vi "LH_InsertAheadIndex.vi"(1 "Index":i32, 2 "InsertContent":i32, 3 "InputList":refnum<class "ListHead.lvclass">) -> (0 "OutputList":refnum<class "ListHead.lvclass">)   [LabVIEW 2014, in "ListHead.lvclass"]
uses:
  ListHead.lvclass
  ListHead.lvclass/ListHead.ctl
  ListNode.lvclass
  ListNodeVirtual.lvclass
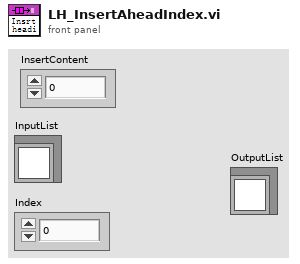
[diagram p1: front panel]
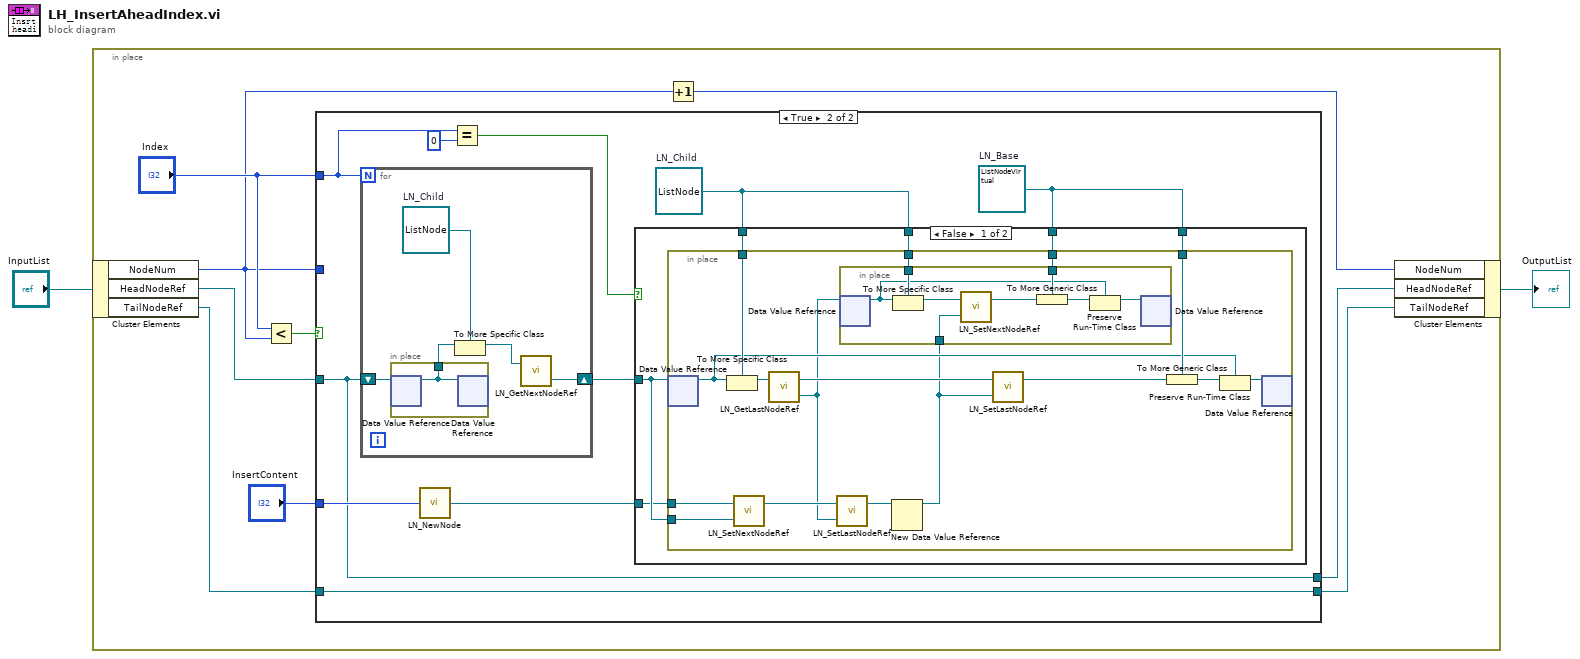
[diagram p0: block diagram]
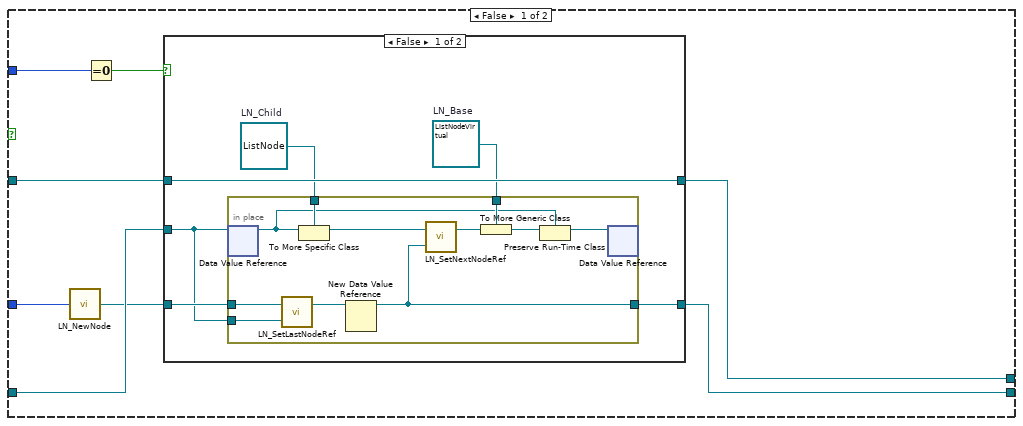
[diagram p2: hidden frame]
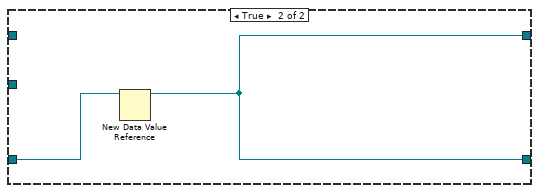
[diagram p3: hidden frame]
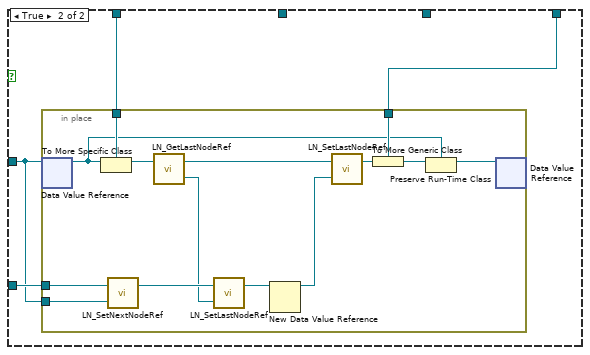
[diagram p4: hidden frame]
diagram:
  n1 = in-place {
    n2 = in-place-cluster #1("InputList") -> ("NodeNum"=w3:u32, "HeadNodeRef"=w9:refnum<data-value>, "TailNodeRef"=w8:refnum<data-value>)
    n3 = Less?(x="Index", y=w3) -> (x < y?=w10:bool)
    n4 = case shown="True" w10 {
      tunnel: w9 -> [w17 w45]
      tunnel: "Index" -> [_ w43]
      tunnel: "InsertContent" -> [w15 w48]
      tunnel: w8 -> [w16 w44]
      tunnel: [w13 w45] -> w5
      tunnel: [w12 w44] -> w4
      tunnel: w3 -> [w19 _]
      frame False {
        n5 = call "LN_NewNode.vi"("InputContent"=w15) -> ("OutputListNode"=w14:refnum<class "ListNode.lvclass">)
        n6 = Equal To 0?(x=w19) -> (x = 0?=w18:bool)
        n7 = case shown="False" w18 {
          tunnel: w14 -> [w23 w38]
          tunnel: w17 -> [w25 _]
          tunnel: w16 -> [w22 _]
          tunnel: [w20 w37] -> w12
          tunnel: [w25 w37] -> w13
          frame False {
            w21 = refnum<class "ListNodeVirtual.lvclass"> refnum  # LN_Base
            w24 = refnum<class "ListNode.lvclass"> refnum  # LN_Child
            n8 = in-place {
              in-place-border: [w27] -> w20
              in-place-border: w24 -> [w36]
              in-place-border: w23 -> [w31]
              in-place-border: w22 -> [w30]
              in-place-border: w21 -> [w35]
              n9 = in-place-dvr #2(w22) -> (w33:refnum<class "ListNodeVirtual.lvclass">)  [unwired: 1 out]
              n10 = call "LN_SetLastNodeRef.vi"("InputLastNodeRef"=w30, "InputListNode"=w31) -> ("OutputListNode"=w29:refnum<class "ListNode.lvclass">)  [unwired: 1 in]
              n11 = To More Specific Class(target class=w36, reference=w33) -> (specific class reference=w28:refnum<class "ListNode.lvclass">)  [unwired: 1 in, 1 out]
              n12 = New Data Value Reference(data value=w29) -> (data value reference=w27:refnum<data-value>)  [unwired: 1 in, 1 out]
              n13 = call "LN_SetNextNodeRef.vi"("InputNextNodeRef"=w27, "InputListNode"=w28) -> ("OutputListNode"=w26:refnum<class "ListNode.lvclass">)  [unwired: 1 in]
              n14 = To More Generic Class(target class=w35, reference=w26) -> (generic class reference=w34:refnum<class "ListNodeVirtual.lvclass">)
              n15 = Preserve Run-Time Class(object in=w34, 2:w33) -> (object out=w32:refnum<class "ListNodeVirtual.lvclass">)  [unwired: 1 in, 1 out]
              n16 = in-place-dvr #2(w32) -> ()  [unwired: 2 out]
            }
          }
          frame True {
            n17 = New Data Value Reference(data value=w38) -> (data value reference=w37:refnum<data-value>)  [unwired: 1 in, 1 out]
          }
        }
      }
      frame True {
        w39 = refnum<class "ListNodeVirtual.lvclass"> refnum  # LN_Base
        w40 = refnum<class "ListNode.lvclass"> refnum  # LN_Child
        n18 = for {
          N: w43 -> [_]
          shift-right: [w97] -> w46
          shift-left: w45 -> [w101]
          w100 = refnum<class "ListNode.lvclass"> refnum  # LN_Child
          n19 = in-place {
            in-place-border: [w102] -> w99
            n20 = in-place-dvr #3(w101) -> (w102:refnum<class "ListNodeVirtual.lvclass">)  [unwired: 1 out]
            n21 = in-place-dvr #3(w102) -> ()  [unwired: 2 out]
          }
          n22 = To More Specific Class(target class=w100, reference=w99) -> (specific class reference=w98:refnum<class "ListNode.lvclass">)  [unwired: 1 in, 1 out]
          n23 = call "LN_GetNextNodeRef.vi"("InputListNode"=w98) -> ("OutputNextNodeRef"=w97:refnum<data-value>)  [unwired: 1 in, 1 out]
        }
        n24 = call "LN_NewNode.vi"("InputContent"=w48) -> ("OutputListNode"=w47:refnum<class "ListNode.lvclass">)
        n25 = Equal?(x=w43, y=0) -> (x = y?=w41:bool)
        n26 = case shown="False" w41 {
          tunnel: w40 -> [w52 w82]
          tunnel: w47 -> [w53 w81]
          tunnel: w46 -> [w54 w80]
          tunnel: w39 -> [w51 w79]
          tunnel: w40 -> [w50 _]
          tunnel: w39 -> [w49 _]
          frame False {
            n27 = in-place {
              in-place-border: w52 -> [w70]
              in-place-border: w53 -> [w62]
              in-place-border: w54 -> [w61]
              in-place-border: w51 -> [w69]
              in-place-border: w50 -> [w57]
              in-place-border: w49 -> [w55]
              n28 = in-place-dvr #4(w54) -> (w67:refnum<class "ListNodeVirtual.lvclass">)  [unwired: 1 out]
              n29 = To More Specific Class(target class=w70, reference=w67) -> (specific class reference=w65:refnum<class "ListNode.lvclass">)  [unwired: 1 in, 1 out]
              n30 = call "LN_SetNextNodeRef.vi"("InputNextNodeRef"=w61, "InputListNode"=w62) -> ("OutputListNode"=w60:refnum<class "ListNode.lvclass">)  [unwired: 1 in]
              n31 = call "LN_GetLastNodeRef.vi"("InputListNode"=w65) -> ("OutputLastNodeRef"=w58:refnum<data-value>, "OutputListNode"=w64:refnum<class "ListNode.lvclass">)  [unwired: 1 in]
              n32 = call "LN_SetLastNodeRef.vi"("InputLastNodeRef"=w58, "InputListNode"=w60) -> ("OutputListNode"=w59:refnum<class "ListNode.lvclass">)  [unwired: 1 in]
              n33 = New Data Value Reference(data value=w59) -> (data value reference=w56:refnum<data-value>)  [unwired: 1 in, 1 out]
              n34 = in-place {
                in-place-border: w57 -> [w77]
                in-place-border: w56 -> [w76]
                in-place-border: w55 -> [w74]
                n35 = in-place-dvr #5(w58) -> (w72:refnum<class "ListNodeVirtual.lvclass">)  [unwired: 1 out]
                n36 = To More Specific Class(target class=w77, reference=w72) -> (specific class reference=w78:refnum<class "ListNode.lvclass">)  [unwired: 1 in, 1 out]
                n37 = call "LN_SetNextNodeRef.vi"("InputNextNodeRef"=w76, "InputListNode"=w78) -> ("OutputListNode"=w75:refnum<class "ListNode.lvclass">)  [unwired: 1 in]
                n38 = To More Generic Class(target class=w74, reference=w75) -> (generic class reference=w73:refnum<class "ListNodeVirtual.lvclass">)
                n39 = Preserve Run-Time Class(object in=w73, 2:w72) -> (object out=w71:refnum<class "ListNodeVirtual.lvclass">)  [unwired: 1 in, 1 out]
                n40 = in-place-dvr #5(w71) -> ()  [unwired: 2 out]
              }
              n41 = call "LN_SetLastNodeRef.vi"("InputLastNodeRef"=w56, "InputListNode"=w64) -> ("OutputListNode"=w63:refnum<class "ListNode.lvclass">)  [unwired: 1 in]
              n42 = To More Generic Class(target class=w69, reference=w63) -> (generic class reference=w68:refnum<class "ListNodeVirtual.lvclass">)
              n43 = Preserve Run-Time Class(object in=w68, 2:w67) -> (object out=w66:refnum<class "ListNodeVirtual.lvclass">)  [unwired: 1 in, 1 out]
              n44 = in-place-dvr #4(w66) -> ()  [unwired: 2 out]
            }
          }
          frame True {
            n45 = in-place {
              in-place-border: w82 -> [w96]
              in-place-border: w81 -> [w87]
              in-place-border: w80 -> [w86]
              in-place-border: w79 -> [w95]
              n46 = in-place-dvr #6(w80) -> (w93:refnum<class "ListNodeVirtual.lvclass">)  [unwired: 1 out]
              n47 = To More Specific Class(target class=w96, reference=w93) -> (specific class reference=w91:refnum<class "ListNode.lvclass">)  [unwired: 1 in, 1 out]
              n48 = call "LN_SetNextNodeRef.vi"("InputNextNodeRef"=w86, "InputListNode"=w87) -> ("OutputListNode"=w85:refnum<class "ListNode.lvclass">)  [unwired: 1 in]
              n49 = call "LN_GetLastNodeRef.vi"("InputListNode"=w91) -> ("OutputLastNodeRef"=w84:refnum<data-value>, "OutputListNode"=w90:refnum<class "ListNode.lvclass">)  [unwired: 1 in]
              n50 = call "LN_SetLastNodeRef.vi"("InputLastNodeRef"=w84, "InputListNode"=w85) -> ("OutputListNode"=w83:refnum<class "ListNode.lvclass">)  [unwired: 1 in]
              n51 = New Data Value Reference(data value=w83) -> (data value reference=w88:refnum<data-value>)  [unwired: 1 in, 1 out]
              n52 = call "LN_SetLastNodeRef.vi"("InputLastNodeRef"=w88, "InputListNode"=w90) -> ("OutputListNode"=w89:refnum<class "ListNode.lvclass">)  [unwired: 1 in]
              n53 = To More Generic Class(target class=w95, reference=w89) -> (generic class reference=w94:refnum<class "ListNodeVirtual.lvclass">)
              n54 = Preserve Run-Time Class(object in=w94, 2:w93) -> (object out=w92:refnum<class "ListNodeVirtual.lvclass">)  [unwired: 1 in, 1 out]
              n55 = in-place-dvr #6(w92) -> ()  [unwired: 2 out]
            }
          }
        }
      }
    }
    n56 = Increment(x=w3) -> (x+1=w6:u32)
    n57 = in-place-cluster #1("NodeNum"=w6, "HeadNodeRef"=w5, "TailNodeRef"=w4) -> (→"OutputList":refnum<class "ListHead.lvclass">)
  }
